vi "convert end of line.vi"(10 "XML":string) -> (2 "String":string)   [LabVIEW 2018, in "Serializer.lvclass"]
uses:
  Serializer.lvclass
  <userlib>/_OpenG.lib/string/string.llb/Convert EOLs (String)__ogtk.vi
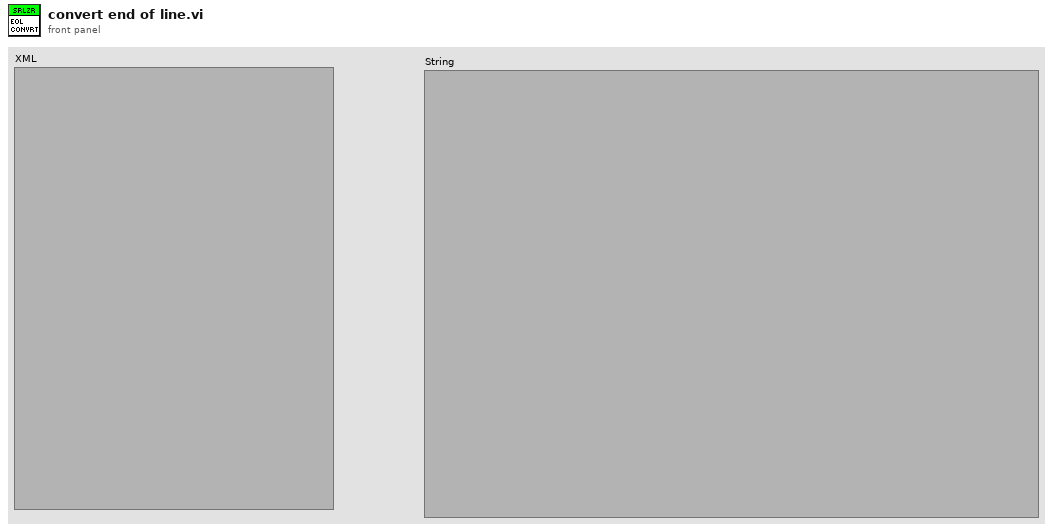
[diagram p1: front panel]
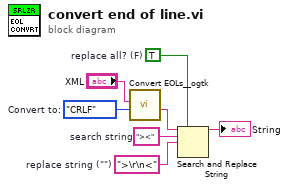
[diagram p0: block diagram]
diagram:
  w2 = TRUE  # replace all? (F)
  w3 = "><"  # search string
  w4 = ">\r\n<"  # replace string ("")
  w6 = enum16{"CR", "LF", "CRLF"}."CRLF"  # Convert to:
  n1 = call-poly <userlib>:"Convert EOLs__ogtk.vi"("Convert to:"=w6, "String in"="XML") -> ("String out"=w5:string)  [unwired: 9 in]
  n2 = Search and Replace String(replace all?=w2, input string=w5, search string=w3, replace string=w4) -> (result string=→"String":string)  [unwired: 4 in, 3 out]
